vi "Three-ENC_Test.vi"() -> ()   [LabVIEW 2019]
panel:
  out "Counter Value":dbl[](array[numeric]) format="%.2f"
  in  "Reset":bool[](array[boolean])
  in  "Error In":errorcluster
  out "Error Out":errorcluster
  in  "Stop":bool
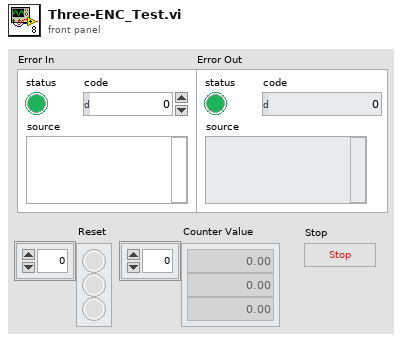
[diagram p1: front panel]
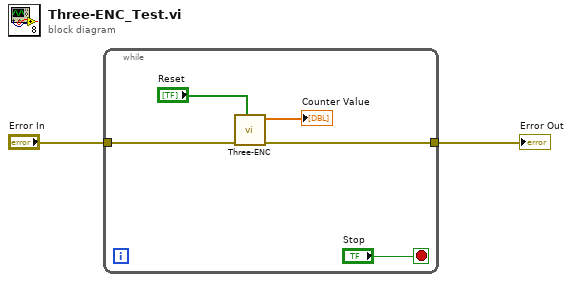
[diagram p0: block diagram]
diagram:
  n1 = while {
    tunnel: [w6] -> w2
    tunnel: "Error In" -> [w5]
    stop <- "Stop" stop-if-true
    n2 = call "Three-ENC.vi"("Reset"="Reset", "Error In"=w5) -> ("Error Out"=w6:errorcluster, "Counter Value"=→"Counter Value":dbl[])  [unwired: 8 in]
  }
  "Error Out" <- w2
